vi "SubConfocal_GetShutterStatus.vi"(7 "Confocal scanner":T1={"SDC shutter"=FALSE, "FWPosition"=2, "FW speed"=3, "Disk spinning?"=FALSE, "Disk speed (rpm)"=4000.0, "Actual speed (rpm)"="0"} {"Disk speed (rpm)" min=1500.0 max=10000.0; "FW speed" min=1 max=3 step=1; "FWPosition" items=["CFP"=1, "GFP"=2, "mCherry"=3, "Alexa647"=4, "OFP"=5, "- empty 6 -"=6]}, 8 "Error In":errorcluster, 11 "Confocal line (VISA In)":refnum<visa-resource-name>="COM1") -> (0 "Error out":errorcluster, 3 "VISA OUT":refnum<visa-resource-name>)   [LabVIEW 2015]
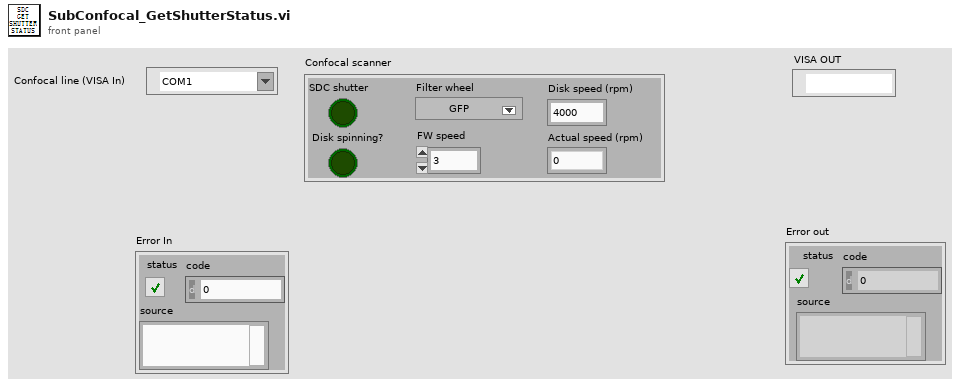
[diagram p1: front panel]
types:
  T1 = cluster{"SDC shutter":bool, "FWPosition":i32, "FW speed":i32, "Disk spinning?":bool, "Disk speed (rpm)":dbl, "Actual speed (rpm)":string}
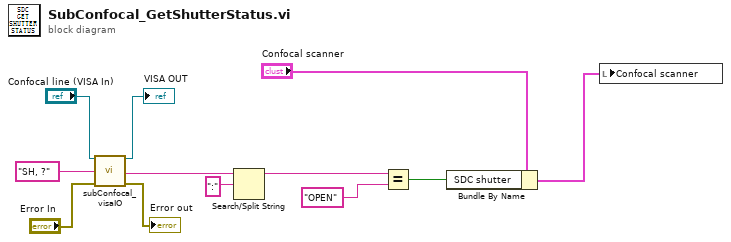
[diagram p0: block diagram]
diagram:
  n1 = call "subConfocal_visaIO.vi"("VISA  IN"="Confocal line (VISA In)", "Command (to ctlr)"="SH, ?", "error in"="Error In") -> ("VISA OUT"=→"VISA OUT":refnum<visa-resource-name>, "Raw Response"=w7:string, "error out"=→"Error out":errorcluster)  [unwired: 8 in, 2 out]
  n2 = Search/Split String(string=w7, search string/char (-)=":") -> (substring before match=w5:string)  [unwired: 1 in, 2 out]
  n3 = Equal?(x=w5, y="OPEN") -> (x = y?=w3:bool)
  n4 = Bundle By Name(cluster="Confocal scanner", "SDC shutter"=w3) -> (w1:T1)
  n5 = local write "Confocal scanner"(w1) -> ()
